vi "PID Error.vi"(10 "Setpoint":dbl, 11 "Position":dbl) -> (3 "Error":dbl)   [LabVIEW 2014]
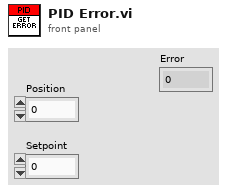
[diagram p1: front panel]
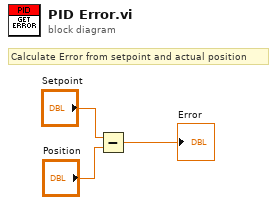
[diagram p0: block diagram]
diagram:
  # "Calculate Error from setpoint and actual position"
  n1 = Subtract(x="Setpoint", y="Position") -> (x-y=→"Error":dbl)
